vi "Resize Vertical Toolbar Dialog.vi"(6 "Mouse Position":cluster{"Horizontal":i32, "Vertical":i32}, 7 "Border Size":i16, 8 "error in (no error)":errorcluster, 9 "Draw Area Size":cluster{"Width":u32, "Height":u32}={"Width"=162, "Height"=720}, 10 "2D Picture Ref":refnum<vi>, 11 "Dialog VI Ref":refnum<vi>) -> (0 "error out":errorcluster)   [LabVIEW 2011, in "Toolbar Control.lvclass"]
doc: "This VI will resize the Vertical Toolbar Dialog, to have it fit in the screen, and show scrollbars if needed. Provide the <B>Dialog VI Ref</B> and the <B>2D Picture Ref</B> from the dialog VI along with the <B>Border Size</B>, <B>Mouse Position</B> which defines where to put the dialog, and the <B>Draw Area Size</B> which is the size of the vertical toolbar.\n\n-------------\nDeveloped by Brian Hoover (hooovahh)"
uses:
  Toolbar Control.lvclass
  <vilib>/Utility/miscctls.llb/LVRectTypeDef.ctl
  <vilib>/Utility/miscctls.llb/LVBoundsTypeDef.ctl
  <vilib>/Utility/miscctls.llb/LVPointTypeDef.ctl
  <vilib>/Utility/miscctls.llb/LVPositionTypeDef.ctl
  Non Class Utilities/Get Window HWnd.vi
  Non Class Utilities/Set Window Z-Position (hwnd).vi
  <userlib>/_OpenG.lib/error/error.llb/Build Error Cluster__ogtk.vi
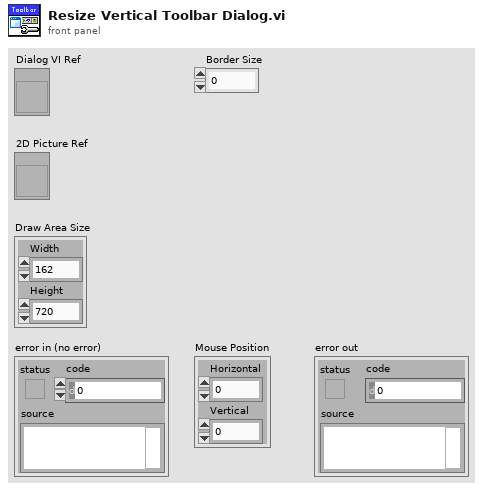
[diagram p1: front panel]
types:
  T1 = typedef "LVPositionTypeDef.ctl" = cluster{"Left":i32, "Top":i32}
  T2 = typedef "LVPointTypeDef.ctl" = cluster{"Horizontal":i16, "Vertical":i16}
  T3 = typedef "LVBoundsTypeDef.ctl" = cluster{"Width":u32, "Height":u32}
  T4 = enum16{"Always On", "Always Off", "Off While Running"}
  T5 = typedef "LVRectTypeDef.ctl" = cluster{"Left":i16, "Top":i16, "Right":i16, "Bottom":i16}
  T6 = typedef "LVAllMonitorsDisplayTypeDef.ctl" = cluster{"Bounds":cluster{"Left":i16, "Top":i16, "Right":i16, "Bottom":i16}, "Depth":i16}[]
  T7 = cluster{"Left":i16, "Top":i16, "Right":i16, "Bottom":i16}
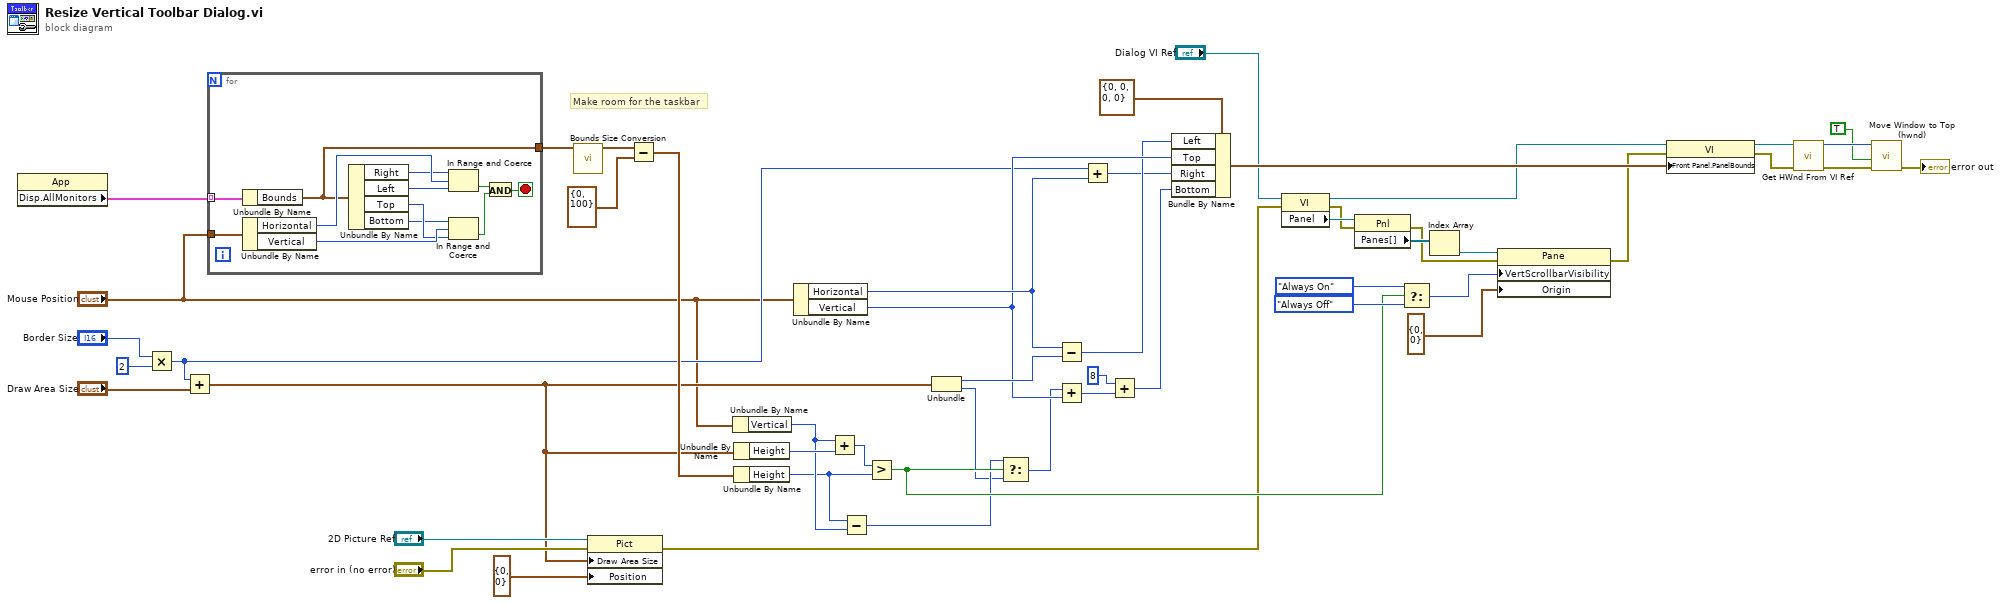
[diagram p0: block diagram]
diagram:
  # "Make room for the taskbar"
  n1 = property class="App"() -> ("Disp.AllMonitors"=w51:T6)  [unwired: 2 in, 2 out]
  n2 = Multiply(x="Border Size", y=i16 2) -> (x*y=w10:i16)
  n3 = Add(x=w10, y="Draw Area Size") -> (x+y=w11:cluster{"Width":u32, "Height":u32})
  n4 = for {
    tunnel: w51 -> [w53] mode=indexing
    tunnel: "Mouse Position" -> [w63]
    tunnel: [w52] -> w50
    stop <- w54 stop-if-true
    n5 = Unbundle By Name(w53) -> ("Bounds"=w52:T7)
    n6 = Unbundle By Name(w63) -> ("Horizontal"=w62:i32, "Vertical"=w61:i32)
    n7 = Unbundle By Name(w52) -> ("Right"=w59:i16, "Left"=w60:i16, "Top"=w58:i16, "Bottom"=w57:i16)
    n8 = In Range and Coerce(upper limit=w59, x=w62, lower limit=w60) -> (In Range?=w55:bool)  [unwired: 1 out]
    n9 = In Range and Coerce(upper limit=w57, x=w61, lower limit=w58) -> (In Range?=w56:bool)  [unwired: 1 out]
    n10 = And(x=w55, y=w56) -> (x .and. y?=w54:bool)
  }
  n11 = call "Bounds Size Conversion.vi"("Bounds"=w50) -> ("Size Out"=w33:T3)  [unwired: 9 in, 1 out]
  n12 = property on="Property Node" class="Pict"(reference="2D Picture Ref", error in="error in (no error)", "Draw Area Size"=w11, "Position"=T1 {"Left"=0, "Top"=0}) -> (error out=w17:errorcluster)  [unwired: 1 out]
  n13 = Subtract(x=w33, y=T3 {"Width"=0, "Height"=100}) -> (x-y=w32:T3)
  n14 = Unbundle By Name("Mouse Position") -> ("Vertical"=w29:i32)
  n15 = Unbundle By Name(w11) -> ("Height"=w44:u32)
  n16 = Unbundle By Name(w32) -> ("Height"=w28:u32)
  n17 = Unbundle By Name("Mouse Position") -> ("Horizontal"=w48:i32, "Vertical"=w46:i32)
  n18 = Add(x=w29, y=w44) -> (x+y=w43:u32)
  n19 = Subtract(x=w28, y=w29) -> (x-y=w26:u32)
  n20 = Greater?(x=w43, y=w28) -> (0:w27:bool)
  n21 = Unbundle(w11) -> ("Width"=w47:u32, "Height"=w25:u32)
  n22 = Select(t=w26, s=w27, f=w25) -> (s? t:f=w24:u32)
  n23 = Subtract(x=w48, y=w47) -> (x-y=w15:u32)
  n24 = Add(x=w24, y=w46) -> (x+y=w45:u32)
  n25 = Add(x=w10, y=w48) -> (x+y=w14:i32)
  n26 = Add(x=u32 8, y=w45) -> (x+y=w9:u32)
  n27 = Bundle By Name(cluster=T5 {"Left"=0, "Top"=0, "Right"=0, "Bottom"=0} ("Front Panel Window:Panel Bounds"), "Left"=w15, "Top"=w46, "Right"=w14, "Bottom"=w9) -> (w31:T5)
  n28 = property class="VI"(reference="Dialog VI Ref", error in=w17) -> (reference out=w16:refnum<vi>, error out=w39:errorcluster, "Panel"=w42:refnum<vi>)
  n29 = property class="Pnl"(reference=w42, error in=w39) -> (error out=w38:errorcluster, "Panes[]"=w41:refnum<vi>[])  [unwired: 1 out]
  n30 = Select(t=T4."Always On" ("Vertical Scrollbar Visibility"), s=w27, f=T4."Always Off" ("Vertical Scrollbar Visibility")) -> (s? t:f=w35:T4)
  n31 = Index Array(array=w41) -> (element=w40:refnum<vi>)  [unwired: 1 in]
  n32 = property class="Pane"(reference=w40, error in=w38, "VertScrollbarVisibility"=w35, "Origin"=T2 {"Horizontal"=0, "Vertical"=0}) -> (error out=w30:errorcluster)  [unwired: 1 out]
  n33 = property class="VI"(reference=w16, error in=w30, "Front Panel.PanelBounds"=w31) -> (reference out=w7:refnum<vi>, error out=w3:errorcluster)
  n34 = call "Get HWnd From VI Ref.vi"("error in (no error)"=w3, "VI reference (calling VI)"=w7) -> ("error out"=w4:errorcluster, "HWnd Out"=w6:u32)  [unwired: 8 in]
  n35 = call "Move Window to Top (hwnd).vi"("error in (no error)"=w4, "Activate? (F)"=TRUE, "HWnd"=w6) -> ("error out"=→"error out":errorcluster)  [unwired: 7 in, 1 out]
